vi "Homing_KCubeDCServo.vi"(9 "Homing type":enum16{"Custom Homing", "Kinesis Homing"}(ring), 10 "set absolute position":dbl, 11 ".NET Refnum in":refnum<k24>) -> (1 "Direction":i32(ring)=1 items=["Clockwise"=1, "CounterClockwise"=2], 3 "Homing":bool)   [LabVIEW 2019]
doc: "set custom or Kinesis-style homing for DC servo motor"
uses:
  D:/Victor Sun/optical trap control/Kinesis/ThorLabs.MotionControl.KCube.DCServoCLI.dll
  Kinesis/ThorLabs.MotionControl.KCube.DCServoCLI.dll
  D:/Victor Sun/optical trap control/Kinesis/Thorlabs.MotionControl.GenericMotorCLI.dll
  Kinesis/Thorlabs.MotionControl.GenericMotorCLI.dll
panel:
  out "Velocity":dbl
  out "LimitSwitch":i32(ring) items=["Ignore"=0, "ClockwiseHard"=1, "CounterClockwiseHard"=4]
  out "OffsetDistance":dbl
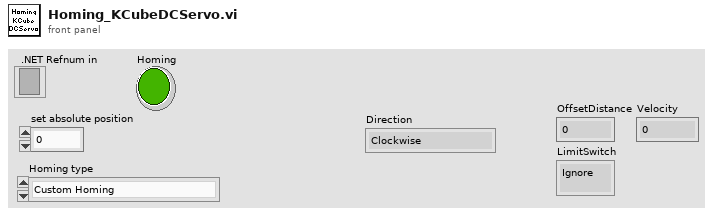
[diagram p1: front panel]
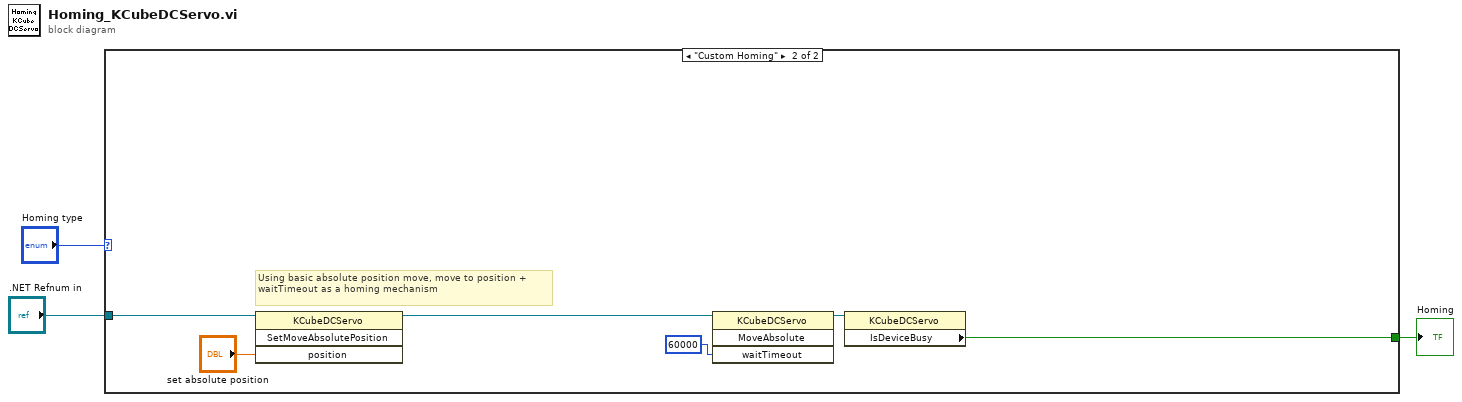
[diagram p0: block diagram]
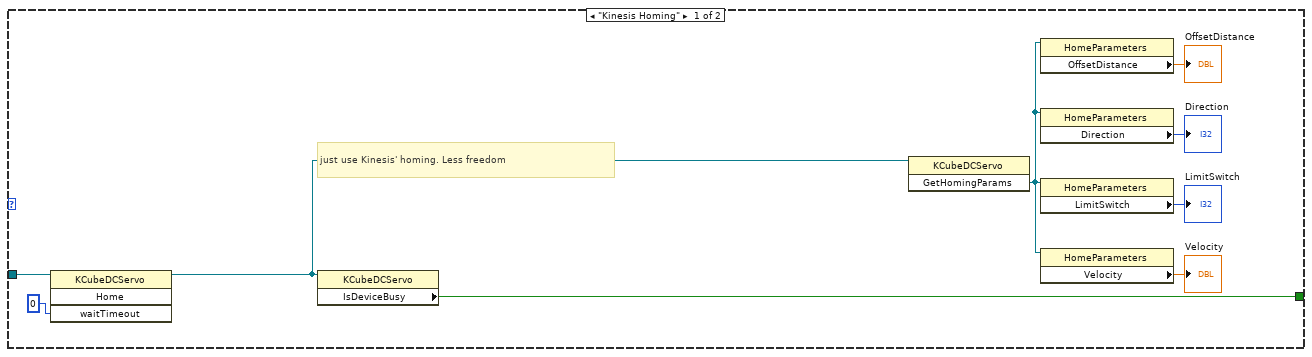
[diagram p2: hidden frame]
diagram:
  n1 = case shown="\"Custom Homing\"" "Homing type" {
    tunnel: ".NET Refnum in" -> [w12 w14]
    tunnel: [w11 w13] -> w1
    frame "Kinesis Homing" {
      # "just use Kinesis' homing. Less freedom"
      n2 = invoke class="KCubeDCServo" method="Home"(reference=w12, "waitTimeout"=0) -> (reference out=w6:refnum<k24>)  [unwired: 2 in, 3 out]
      n3 = property class="KCubeDCServo"(reference=w6) -> ("IsDeviceBusy"=w11:bool)  [unwired: 1 in, 2 out]
      n4 = invoke class="KCubeDCServo" method="GetHomingParams"(reference=w6) -> ("GetHomingParams"=w4:refnum<k24>)  [unwired: 2 in, 2 out]
      n5 = property class="HomeParameters"(reference=w4) -> ("OffsetDistance"=→"OffsetDistance":dbl)  [unwired: 1 in, 2 out]
      n6 = property class="HomeParameters"(reference=w4) -> ("Direction"=→"Direction":i32)  [unwired: 1 in, 2 out]
      n7 = property class="HomeParameters"(reference=w4) -> ("LimitSwitch"=→"LimitSwitch":i32)  [unwired: 1 in, 2 out]
      n8 = property class="HomeParameters"(reference=w4) -> ("Velocity"=→"Velocity":dbl)  [unwired: 1 in, 2 out]
    }
    frame "Custom Homing" {
      # "Using basic absolute position move, move to position + waitTimeout as a homing mechanism"
      n9 = invoke class="KCubeDCServo" method="SetMoveAbsolutePosition"(reference=w14, "position"="set absolute position") -> (reference out=w15:refnum<k24>)  [unwired: 2 in, 3 out]
      n10 = invoke class="KCubeDCServo" method="MoveAbsolute"(reference=w15, "waitTimeout"=60000) -> (reference out=w18:refnum<k24>)  [unwired: 2 in, 3 out]
      n11 = property class="KCubeDCServo"(reference=w18) -> ("IsDeviceBusy"=w13:bool)  [unwired: 1 in, 2 out]
    }
  }
  "Homing" <- w1
